vi "Query Word.vi"(8 "error in (no error)":errorcluster, 10 "Query String":string, 11 "BH Druck PACE Series in":refnum<class "BH Druck PACE Series.lvclass">) -> (0 "error out":errorcluster, 2 "String Result":string, 3 "BH Druck PACE Series out":refnum<class "BH Druck PACE Series.lvclass">)   [LabVIEW 2022 SP3, in "BH Druck PACE Series.lvclass"]
uses:
  BH Druck PACE Series.lvclass
  BH Druck PACE Series.lvclass/BH Druck PACE Series.ctl
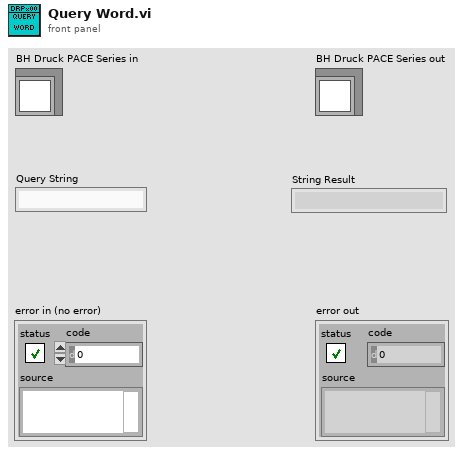
[diagram p1: front panel]
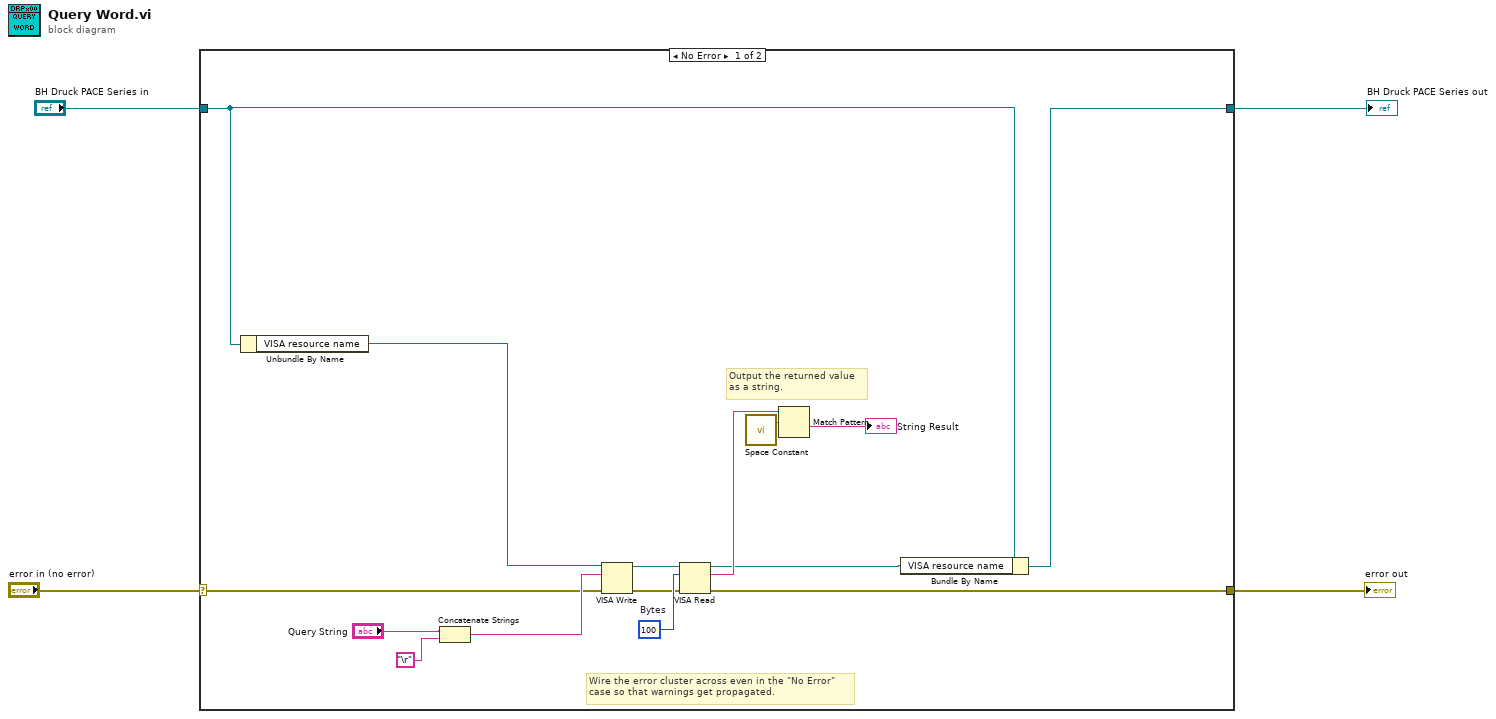
[diagram p0: block diagram]
diagram:
  n1 = case shown="No Error" "error in (no error)" {
    selector: "error in (no error)" -> [w10 w21]
    tunnel: [w9 w21] -> w3
    tunnel: [w5 w20] -> w1
    tunnel: "BH Druck PACE Series in" -> [w6 w20]
    frame No Error {
      w19 = u32 100  # Bytes
      # "Output the returned value\nas a string."
      # "Wire the error cluster across even in the \"No Error\"\ncase so that warnings get propagated."
      n2 = Unbundle By Name(w6) -> ("VISA resource name"=w8:refnum<visa-resource-name>)
      n3 = Concatenate Strings("Query String", "\r" ("Carriage Return Constant")) -> (w12:string)
      n4 = VISA Write(VISA resource name=w8, write buffer=w12, error in (no error)=w10) -> (VISA resource name out=w18:refnum<visa-resource-name>, error out=w17:errorcluster)  [unwired: 1 out]
      n5 = VISA Read(VISA resource name=w18, byte count=w19, error in (no error)=w17) -> (VISA resource name out=w7:refnum<visa-resource-name>, read buffer=w15:string, error out=w9:errorcluster)  [unwired: 1 out]
      n6 = call <vilib>:"Space Constant.vi"() -> ("String"=w16:string)
      n7 = Match Pattern(string=w15, regular expression=w16) -> (after substring=→"String Result":string)  [unwired: 1 in, 3 out]
      n8 = Bundle By Name(cluster=w6, "VISA resource name"=w7) -> (w5:refnum<class "BH Druck PACE Series.lvclass">)
    }
    frame Error {
    }
  }
  "error out" <- w3
  "BH Druck PACE Series out" <- w1
